vi "Update latest position.vi"(8 "error in (no error)":errorcluster, 11 "ConfocalStage in":refnum<class "ConfocalStage.lvclass">) -> (0 "error out":errorcluster, 3 "ConfocalStage out":refnum<class "ConfocalStage.lvclass">)   [LabVIEW 2012, in "ConfocalStage.lvclass"]
uses:
  ConfocalStage.lvclass
  ConfocalStage.lvclass/ConfocalStage.ctl
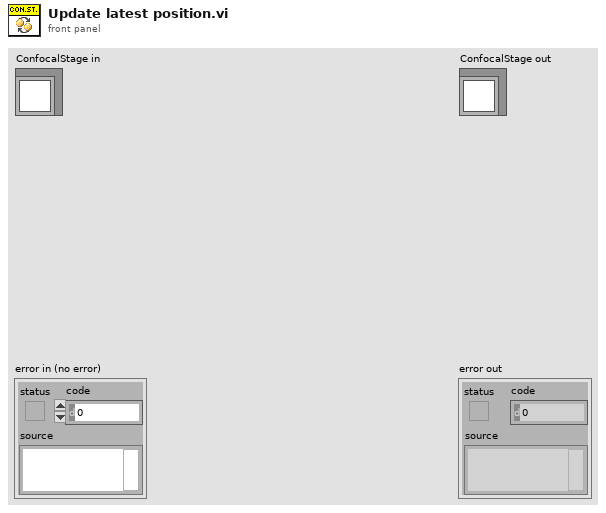
[diagram p1: front panel]
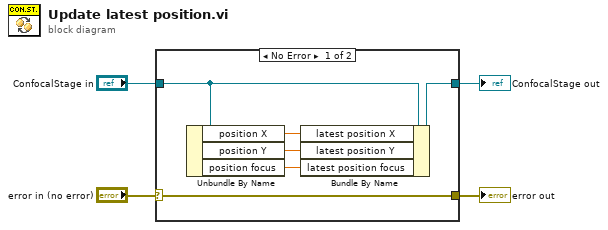
[diagram p0: block diagram]
diagram:
  n1 = case shown="No Error" "error in (no error)" {
    selector: "error in (no error)" -> [w10 w12]
    tunnel: [w10 w12] -> w3
    tunnel: [w8 w11] -> w1
    tunnel: "ConfocalStage in" -> [w9 w11]
    frame No Error {
      n2 = Unbundle By Name(w9) -> ("position X"=w7:dbl, "position Y"=w6:dbl, "position focus"=w5:dbl)
      n3 = Bundle By Name(cluster=w9, "latest position X"=w7, "latest position Y"=w6, "latest position focus"=w5) -> (w8:refnum<class "ConfocalStage.lvclass">)
    }
    frame Error {
    }
  }
  "error out" <- w3
  "ConfocalStage out" <- w1
